vi "Main.vi"(8 "error in (no error)":errorcluster, 11 "ModuleAdmin":refnum<class "ModuleAdmin.lvclass">) -> ()   [LabVIEW 2018, in "MyPlugins.lvlib"]
uses:
  MyPlugins.lvlib
  <userlib>/NIST/ModuleAdminLib/ModuleAdmin/ModuleAdmin.lvclass
  C:/Program Files (x86)/National Instruments/LabVIEW 2018/user.lib/NIST/ModuleAdminLib/ModuleAdminBase/ModuleAdminBase.lvclass
  MyPluginBaseClass/MyPluginsBase.lvclass
  C:/Program Files (x86)/National Instruments/LabVIEW 2018/user.lib/NIST/BaseClasses/BasePlugin_class/BasePlugin.lvclass
  PluginsShared/clStopArgument.ctl
  <userlib>/NIST/ModuleAdminLib/ModuleAdmin/ModuleAdmin.lvclass/ModuleAdmin.ctl
  Queue SubVIs/DequeueTypes.ctl
  <userlib>/NIST/BaseClasses/BasePlugin_class/BasePlugin.lvclass/BasePlugin.ctl
  Queue SubVIs/EnqueueTypes.ctl
  <vilib>/Utility/error.llb/DialogType.ctl
  <userlib>/NIST/ModuleAdminLib/ModuleAdmin/Accessors/Read ShowPanel_.vi
  <userlib>/NIST/ModuleAdminLib/ModuleAdmin/Accessors/Write ShowPanel_.vi
  <userlib>/NIST/BaseClasses/BasePlugin_class/Accessors/Write PluginIniFilePath.vi
  <userlib>/NIST/BaseClasses/BasePlugin_class/Accessors/Read PluginIniFilePath.vi
  <userlib>/NIST/ModuleAdminLib/ModuleAdmin/Accessors/Read CloneRegRef.vi
  <vilib>/Utility/error.llb/Error Cluster From Error Code.vi
  <vilib>/ErrorRing/Error Ring.xnode
  <userlib>/NIST/ModuleAdminLib/CloneRegistration/CloneRegistration.lvclass
  PluginsShared/PluginsShared.lvlib
  <userlib>/NIST/BaseClasses/Object_class/BaseObject.lvclass
  <userlib>/NIST/ModuleAdminLib/ModuleAdmin.lvlib
panel:
  in  "USE FGV?":bool
  out "error out":errorcluster
  # "This is the template for your cloneable module.\nYou should modifiy this to perform the functionality\nthat you want it to perform"
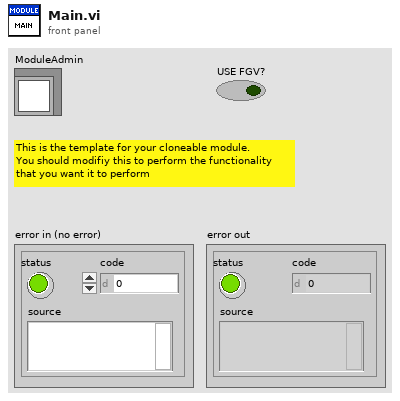
[diagram p1: front panel]
types:
  T1 = typedef "PluginsShared.lvlib/clRequestEvents.ctl" = cluster{"StopRequest":refnum<user-event>, "PathToINI":refnum<user-event>, " LoadPlugin":refnum<user-event>, "ShowPanel":refnum<user-event>, "PrefDlg":refnum<user-event>}
  T2 = typedef "PluginsShared.lvlib/clBroadcastEvents.ctl" = cluster{"DidInit":refnum<user-event>, "StatusUpdate":refnum<user-event>, "ErrorReport":refnum<user-event>, "DidStop":refnum<user-event>, "PathToINI":refnum<user-event>, "ReloadINIFiles":refnum<user-event>}
  T3 = typedef "PluginsShared.lvlib/clStopArgument.ctl" = cluster{"Exit via Stop Module Req?":bool, "Wait for Module to stop?":bool, "ModuleAdmin":refnum<class "ModuleAdmin.lvclass">}
  T4 = enum32{"Invalid", "Standard", "Closed", "Hidden", "Minimized", "Maximized"}
  T5 = typedef "MyPlugins.lvlib/EnqueueTypes.ctl" = enum16{"Enqueue", "Lossy Enqueue"}
  T6 = typedef "MyPlugins.lvlib/DequeueTypes.ctl" = enum16{"Dequeue", "Preview Queue"}
  T7 = typedef "DialogType.ctl" = u16
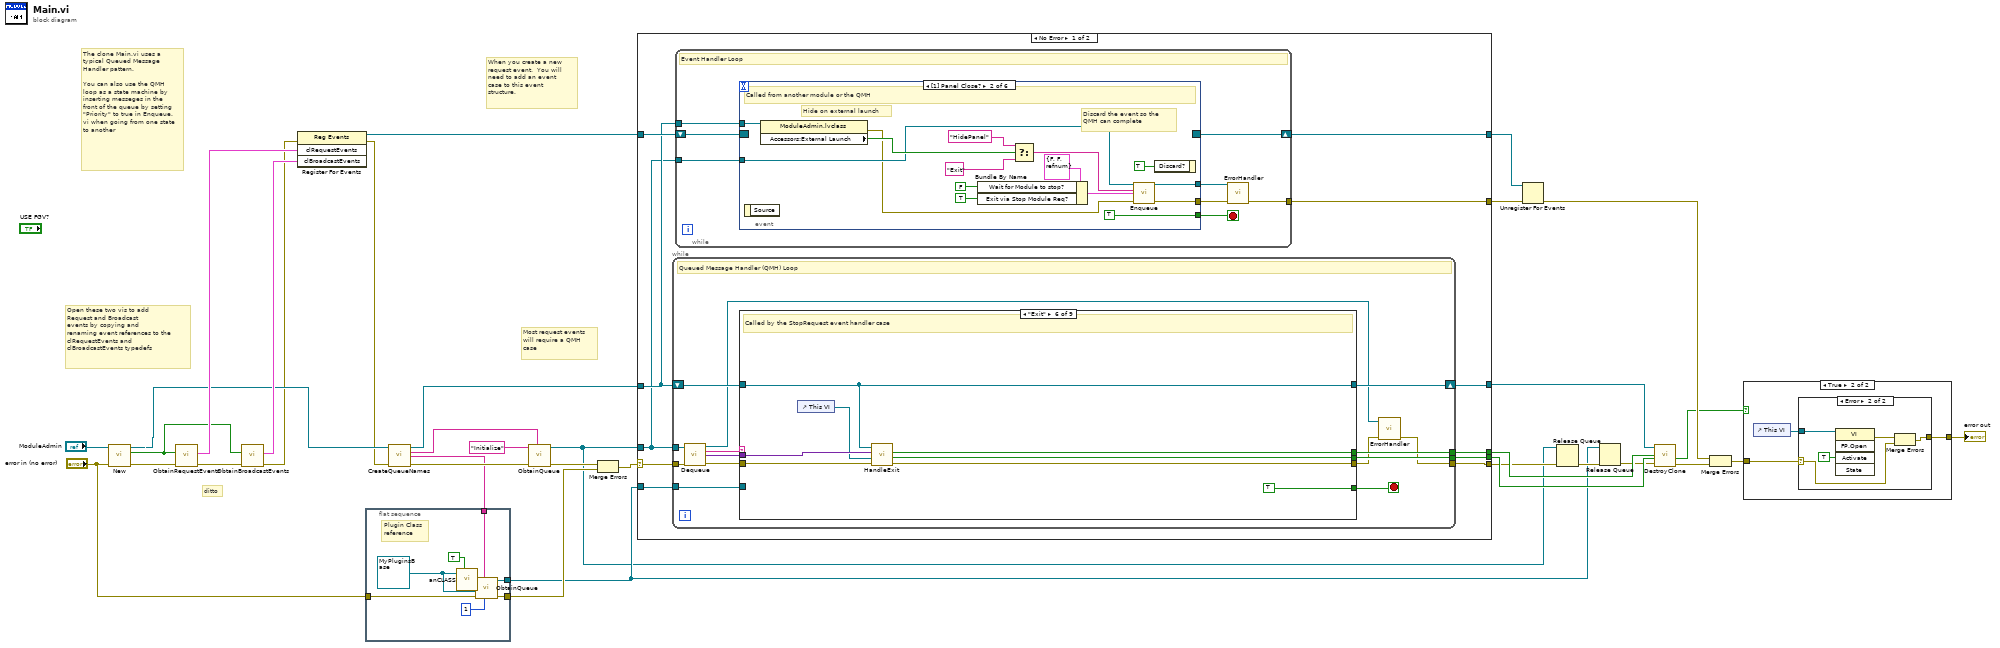
[diagram p0: block diagram]
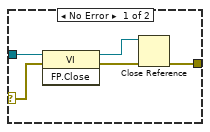
[diagram p3: hidden frame]
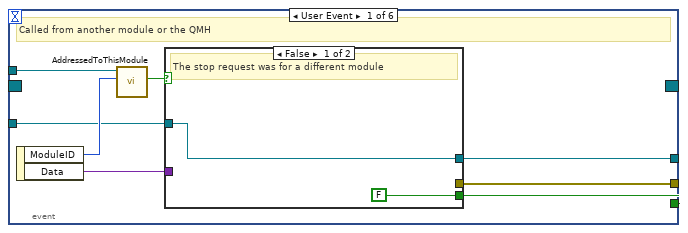
[diagram p4: hidden frame]
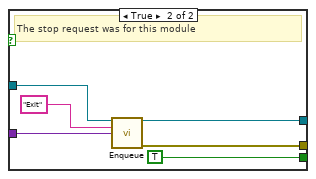
[diagram p5: hidden frame]
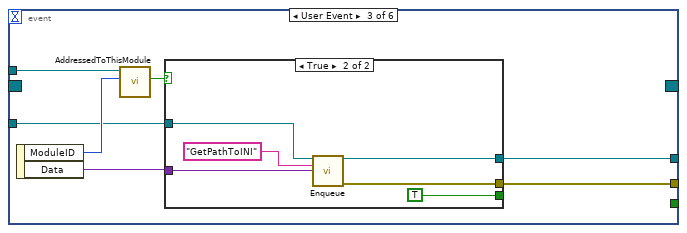
[diagram p6: hidden frame]
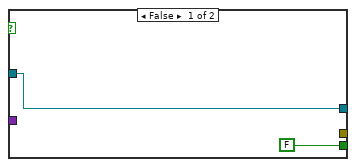
[diagram p7: hidden frame]
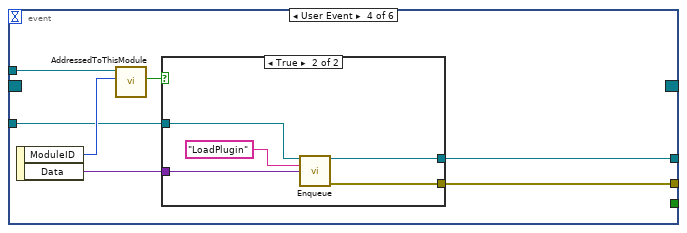
[diagram p8: hidden frame]
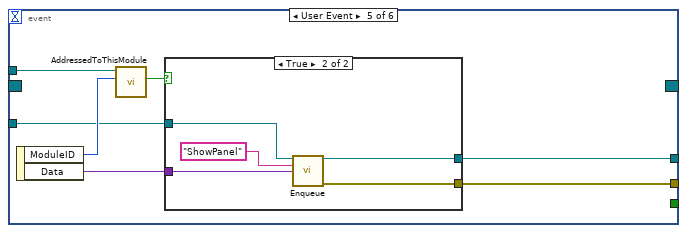
[diagram p10: hidden frame]
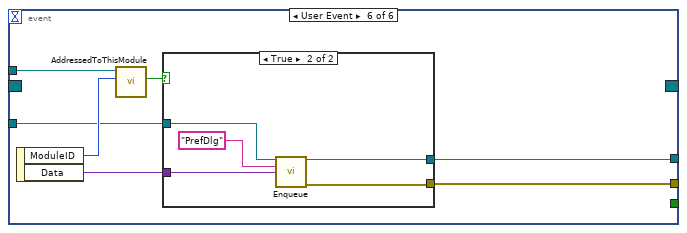
[diagram p12: hidden frame]
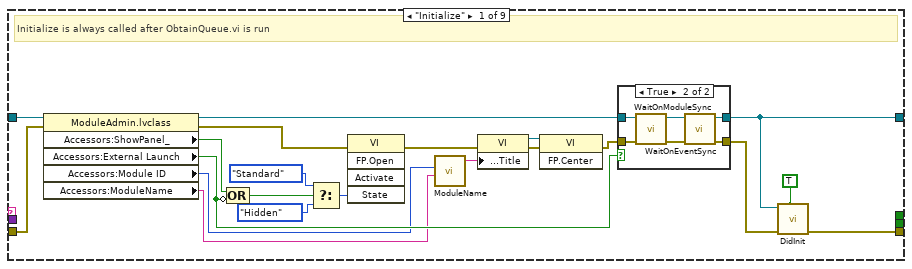
[diagram p14: hidden frame]
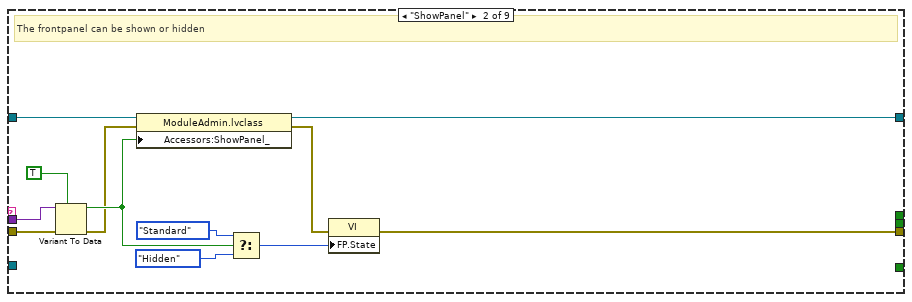
[diagram p16: hidden frame]
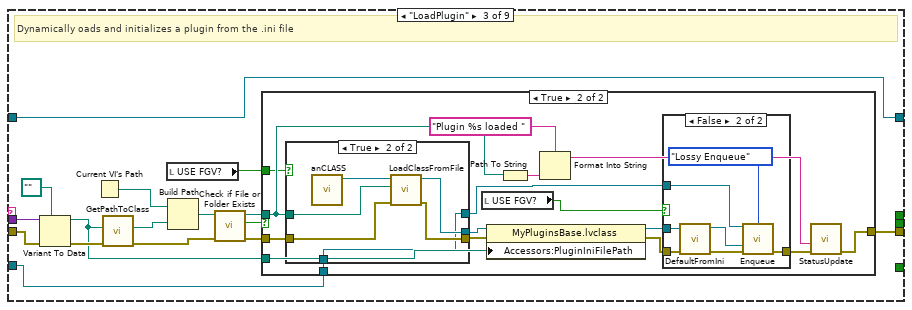
[diagram p17: hidden frame]
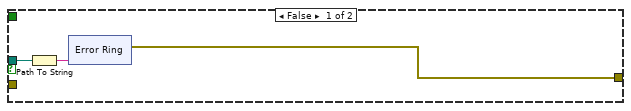
[diagram p18: hidden frame]
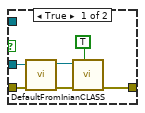
[diagram p19: hidden frame]
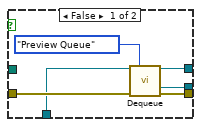
[diagram p20: hidden frame]
diagram:
  # "The clone Main.vi uses a typical Queued Message Handler pattern.  \n\nYou can also use the QMH loop as a state machine by inserting messeges in the front of the queue by setting \"Priority\" to true in Enqueue.vi when going from one state to another"
  # "Open these two vis to add\nRequest and Broadcast \nevents by copying and \nrenaming event references to the \nclRequestEvents and \nclBroadcastEvents typedefs"
  # "ditto"
  # "Most request events\nwill require a QMH\ncase"
  # "When you create a new request event.  You will need to add an event case to this event structure."
  n1 = call <userlib>:"New.vi"("error in (no error)"="error in (no error)", "ModuleAdmin"="ModuleAdmin") -> ("error out"=w25:errorcluster, "First?"=w32:bool, "ModuleAdmin"=w12:refnum<class "ModuleAdmin.lvclass">)  [unwired: 6 in, 1 out]
  n2 = call "ObtainRequestEvents.vi"("error in (no error)"=w25, "CreateNew (F)"=w32) -> ("error out"=w31:errorcluster, "clRequestEvents"=w33:T1)  [unwired: 8 in]
  n3 = call "ObtainBroadcastEvents.vi"("error in (no error)"=w31, "CreateNew? (F)"=w32) -> ("error out"=w6:errorcluster, "clBroadcastEvents"=w30:T2)  [unwired: 8 in]
  n4 = register-events(error in=w6, w33, w30) -> (reference out=w29:refnum<event-registration>, error out=w5:errorcluster)  [unwired: 1 in]
  n5 = flat-sequence {
    tunnel: "error in (no error)" -> [w40]
    tunnel: [w39] -> w22
    tunnel: w8 -> [w38]
    tunnel: [w36] -> w2
    frame #0 {
      w37 = refnum<class "MyPluginsBase.lvclass"> refnum ("MyPlugins.lvlib:MyPluginsBase.lvclass")
      # "Plugin Class\nreference"
      n6 = call "anCLASS.vi"("Set? (f)"=TRUE, "MyPlugins.lvlib In"=w37) -> ()  [unwired: 9 in, 1 out]
      n7 = call "ObtainQueue.vi"("max queue size (-1, unlimited)"=1, "Queue Name"=w38, "Error In"=w40, "MyPluginsClass"=w37) -> ("Error Out"=w39:errorcluster, "queue out"=w36:refnum<queue>)  [unwired: 6 in]
    }
  }
  n8 = call "CreateQueueNames.vi"("ModuleAdmin"=w12, "error in (no error)"=w5) -> ("ModuleAdmin Out"=w10:refnum<class "ModuleAdmin.lvclass">, "QMH Queue Name"=w9:string, "Class Queue Name"=w8:string, "error out"=w11:errorcluster)  [unwired: 9 in, 1 out]
  n9 = call "ObtainQueue.vi"("Queue Name"=w9, "Error In"=w11, "InitialMessage"="Initialize" ("Message")) -> ("Error Out"=w14:errorcluster, "queue out"=w1:refnum<queue>)  [unwired: 7 in]
  n10 = Merge Errors(w14, w22) -> (w23:errorcluster)
  n11 = case shown="No Error" w23 {
    selector: w23 -> [w52 w376]
    tunnel: w10 -> [w45 w369]
    tunnel: [w44 w374] -> w16
    tunnel: w29 -> [w51 w370]
    tunnel: [w50 w373] -> w7
    tunnel: [w49 _] -> w19
    tunnel: [w48 _] -> w18
    tunnel: [w47 _] -> w28
    tunnel: [w46 w370] -> w27
    tunnel: w1 -> [w43 _]
    tunnel: w2 -> [w42 _]
    frame No Error {
      n12 = while {
        tunnel: w52 -> [w158]
        tunnel: [w152] -> w44
        tunnel: [w154] -> w49
        tunnel: [w153] -> w48
        shift-right: [w148] -> w50
        shift-left: w45 -> [w149]
        tunnel: w43 -> [w150]
        tunnel: w42 -> [w147]
        stop <- w159 stop-if-true
        # "Queued Message Handler (QMH) Loop"
        n13 = call "Dequeue.vi"("queue in"=w150, "error in (no error)"=w158) -> ("queue out"=w146:refnum<queue>, "Message"=w156:string, "Message Data"=w155:variant, "error out"=w157:errorcluster)  [unwired: 9 in, 1 out]
        n14 = case shown="\"Exit\"" w156 {
          selector: w156 -> [_ _ _ _ _ _ _ _ w357]
          tunnel: [_ _ _ _ _ TRUE _ TRUE _] -> w159
          tunnel: [w170 w193 w205 w275 w293 w329 w332 w349 w351] -> w151
          tunnel: w157 -> [w164 w200 w214 w273 w295 w328 w340 _ _]
          tunnel: w155 -> [_ w199 w216 _ _ w327 w339 _ _]
          tunnel: [_ _ _ _ _ w325 _ _ _] -> w154
          tunnel: [_ _ _ _ _ w324 _ _ _] -> w153
          tunnel: w149 -> [w161 w192 w201 w270 w291 w323 w331 w345 w355]
          tunnel: [w160 w189 w201 w269 w290 w323 w331 w345 w354] -> w148
          tunnel: w147 -> [_ _ w202 w267 w288 _ _ _ _]
          frame "Initialize" {
            # "Initialize is always called after ObtainQueue.vi is run"
            n15 = property class="ModuleAdmin.lvclass"(reference=w161, error in=w164) -> (reference out=w168:refnum<class "ModuleAdmin.lvclass">, error out=w178:errorcluster, "Accessors:ShowPanel_"=w167:bool, "Accessors:External Launch"=w166:bool, "Accessors:Module ID"=w162:i32, "Accessors:ModuleName"=w163:string)
            n16 = Compound Arithmetic op=OR(w167, invert w166) -> (w165:bool)
            n17 = Select(t=T4."Standard" ("Front Panel Window:State"), s=w165, f=T4."Hidden" ("Front Panel Window:State")) -> (s? t:f=w174:T4)
            n18 = invoke class="VI" method="FP.Open"(error in=w178, "State"=w174) -> (error out=w177:errorcluster)  [unwired: 3 in, 4 out]
            n19 = call <userlib>:"ModuleName.vi"("Name"=w163, "ModuleID"=w162) -> ("ModuleName"=w173:string)  [unwired: 9 in]
            n20 = property class="VI"(error in=w177, "Front Panel.Title"=w173) -> (reference out=w180:refnum<vi>, error out=w179:errorcluster)  [unwired: 1 in]
            n21 = invoke class="VI" method="FP.Center"(reference=w180, error in=w179) -> (error out=w169:errorcluster)  [unwired: 1 in, 2 out]
            n22 = case shown="True" w166 {
              tunnel: [w181 w187] -> w171
              tunnel: [w182 w184] -> w160
              tunnel: w169 -> [w181 w186]
              tunnel: w168 -> [w182 w183]
              frame False {
              }
              frame True {
                n23 = call <userlib>:"WaitOnModuleSync.vi"("error in (no error)"=w186, "ModuleAdmin"=w183) -> ("error out"=w188:errorcluster, "ModuleAdmin"=w185:refnum<class "ModuleAdmin.lvclass">)  [unwired: 8 in]
                n24 = call <userlib>:"WaitOnEventSync.vi"("error in (no error)"=w188, "ModuleAdmin"=w185) -> ("error out"=w187:errorcluster, "ModuleAdmin"=w184:refnum<class "ModuleAdmin.lvclass">)  [unwired: 8 in]
              }
            }
            n25 = call "DidInit.vi"("Init?"=TRUE, "error in (no error)"=w171, "ModuleAdmin"=w160) -> ("error out"=w170:errorcluster)  [unwired: 8 in]
          }
          frame "ShowPanel" {
            # "The frontpanel can be shown or hidden"
            n26 = Variant To Data(error in=w200, type=TRUE, Variant=w199) -> (data=w195:bool, error out=w191:errorcluster)
            n27 = property class="ModuleAdmin.lvclass"(reference=w192, error in=w191, "Accessors:ShowPanel_"=w195) -> (reference out=w189:refnum<class "ModuleAdmin.lvclass">, error out=w190:errorcluster)
            n28 = Select(t=T4."Standard" ("Front Panel Window:State"), s=w195, f=T4."Hidden" ("Front Panel Window:State")) -> (s? t:f=w194:T4)
            n29 = property class="VI"(error in=w190, "FP.State"=w194) -> (error out=w193:errorcluster)  [unwired: 1 in, 1 out]
          }
          frame "LoadPlugin" {
            # "Dynamically oads and initializes a plugin from the .ini file"
            n30 = Variant To Data(error in=w214, type=path "", Variant=w216) -> (data=w204:path, error out=w213:errorcluster)
            n31 = Current VI's Path() -> (path=w211:path)
            n32 = call <userlib>:"GetPathToClass.vi"("error in (no error)"=w213, "configuration file path"=w204) -> ("error IO"=w209:errorcluster, "PathToClass"=w212:path)  [unwired: 8 in]
            n33 = local read "USE FGV?"() -> (w203:bool)
            n34 = Build Path(base path=w211, name or relative path=w212) -> (appended path=w210:path)
            n35 = call <vilib>:"Check if File or Folder Exists.vi"("error in (no error)"=w209, "path"=w210) -> ("error out"=w206:errorcluster, "file or folder exists?"=w208:bool, "dup path"=w207:path)  [unwired: 7 in]
            n36 = case shown="True" w208 {
              tunnel: w207 -> [w218 w236]
              tunnel: w206 -> [_ w242]
              tunnel: [w217 w238] -> w205
              tunnel: w204 -> [_ w234]
              tunnel: w203 -> [_ w230]
              tunnel: w202 -> [_ w229]
              frame False {
                n37 = Path To String(path=w218) -> (string=w219:string)
                n38 = xnode "Error Ring"("parameter 0"=w219) -> ("error out"=w217:errorcluster)
              }
              frame True {
                n39 = case shown="True" w230 {
                  tunnel: w242 -> [w260 w266]
                  tunnel: [w258 w265] -> w237
                  tunnel: w236 -> [_ w264]
                  tunnel: [w259 w263] -> w235
                  tunnel: w229 -> [w257 w261]
                  tunnel: [w255 w261] -> w227
                  frame False {
                    n40 = call "Dequeue.vi"("queue in"=w257, "Dequeue Type"=DequeueTypes."Preview Queue", "error in (no error)"=w260) -> ("queue out"=w255:refnum<queue>, "MyPluginsClass"=w258:refnum<class "MyPluginsBase.lvclass">, "error out"=w259:errorcluster)  [unwired: 8 in, 2 out]
                  }
                  frame True {
                    n41 = call "anCLASS.vi"() -> ("MyPlugins.lvlib Out"=w262:refnum<class "MyPluginsBase.lvclass">)  [unwired: 11 in]
                    n42 = call-dynamic "LoadClassFromFile.vi"("error in (no error)"=w266, "class path"=w264, "reference in"=w262) -> ("error out"=w263:errorcluster, "reference out"=w265:refnum<class "MyPluginsBase.lvclass">)  [unwired: 7 in]
                  }
                }
                n43 = local read "USE FGV?"() -> (w228:bool)
                n44 = property class="MyPluginsBase.lvclass"(reference=w237, error in=w235, "Accessors:PluginIniFilePath"=w234) -> (reference out=w233:refnum<class "MyPluginsBase.lvclass">, error out=w232:errorcluster)
                n45 = Path To String(path=w236) -> (string=w240:string)
                n46 = Format Into String(format string="Plugin %s loaded ", w240) -> (resulting string=w239:string)  [unwired: 2 in, 1 out]
                n47 = case shown="False" w228 {
                  tunnel: w233 -> [w247 w254]
                  tunnel: w232 -> [w246 w253]
                  tunnel: [w245 w250] -> w231
                  tunnel: w227 -> [_ w248]
                  frame True {
                    n48 = call-dynamic "DefaultFromIni.vi"("error in (no error)"=w246, "MyPluginsBase in"=w247) -> ("error out"=w245:errorcluster, "MyPluginsBase out"=w244:refnum<class "MyPluginsBase.lvclass">)  [unwired: 8 in]
                    n49 = call "anCLASS.vi"("Set? (f)"=TRUE, "MyPlugins.lvlib In"=w244) -> ()  [unwired: 9 in, 1 out]
                  }
                  frame False {
                    n50 = call-dynamic "DefaultFromIni.vi"("error in (no error)"=w253, "MyPluginsBase in"=w254) -> ("error out"=w251:errorcluster, "MyPluginsBase out"=w252:refnum<class "MyPluginsBase.lvclass">)  [unwired: 8 in]
                    n51 = call "Enqueue.vi"("queue in"=w248, "Enqueue Type (Enqueue)"=EnqueueTypes."Lossy Enqueue", "MyPluginsClass"=w252, "error in (no error)"=w251) -> ("error out"=w250:errorcluster)  [unwired: 10 in, 1 out]
                  }
                }
                n52 = call "StatusUpdate.vi"("error in (no error)"=w231, "Status"=w239) -> ("error out"=w238:errorcluster)  [unwired: 8 in, 1 out]
              }
            }
          }
          frame "GetPathToINI" {
            # "Broadcast the path to the .ini file"
            n53 = local read "USE FGV?"() -> (w268:bool)
            n54 = case shown="False" w268 {
              tunnel: [w280 w287] -> w274
              tunnel: w273 -> [w279 w285]
              tunnel: [w277 w286] -> w272
              tunnel: w267 -> [_ w282]
              frame True {
                n55 = call "anCLASS.vi"() -> ("MyPlugins.lvlib Out"=w278:refnum<class "MyPluginsBase.lvclass">)  [unwired: 11 in]
                n56 = property class="MyPluginsBase.lvclass"(reference=w278, error in=w279) -> (error out=w277:errorcluster, "Accessors:PluginIniFilePath"=w280:path)  [unwired: 1 out]
              }
              frame False {
                n57 = call "Dequeue.vi"("queue in"=w282, "Dequeue Type"=DequeueTypes."Preview Queue", "error in (no error)"=w285) -> ("MyPluginsClass"=w283:refnum<class "MyPluginsBase.lvclass">, "error out"=w284:errorcluster)  [unwired: 8 in, 3 out]
                n58 = property class="MyPluginsBase.lvclass"(reference=w283, error in=w284) -> (error out=w286:errorcluster, "Accessors:PluginIniFilePath"=w287:path)  [unwired: 1 out]
              }
            }
            n59 = property class="ModuleAdmin.lvclass"(reference=w270, error in=w272) -> (reference out=w269:refnum<class "ModuleAdmin.lvclass">, error out=w271:errorcluster, "Accessors:Module ID"=w276:i32)
            n60 = call "PathToINIBroadcast.vi"("error in (no error)"=w271, "PathToINI"=w274, "ModuleID"=w276) -> ("error out"=w275:errorcluster)  [unwired: 8 in]
          }
          frame "PrefDlg" {
            # "Override Base Class\\PublicMethods\\PrefDialog.vi for user editable preference dialog"
            # "Launch the modal Preferences dialog"
            n61 = local read "USE FGV?"() -> (w289:bool)
            n62 = case shown="False" w289 {
              tunnel: w295 -> [w308 w314]
              tunnel: [w304 w312] -> w294
              tunnel: [w302 w310] -> w292
              tunnel: w288 -> [w307 _]
              frame False {
                n63 = call "Dequeue.vi"("queue in"=w307, "Dequeue Type"=DequeueTypes."Preview Queue", "error in (no error)"=w308) -> ("queue out"=w301:refnum<queue>, "MyPluginsClass"=w297:refnum<class "MyPluginsBase.lvclass">, "error out"=w306:errorcluster)  [unwired: 8 in, 2 out]
                n64 = call-dynamic "PrefDialog.vi"("error in (no error)"=w306, "MyPluginsBase in"=w297) -> ("error out"=w303:errorcluster, "ReloadiniFiles"=w304:bool, "ChangeOccured?"=w299:bool, "MyPluginsBase out"=w298:refnum<class "MyPluginsBase.lvclass">)  [unwired: 6 in]
                n65 = Select(t=w298, s=w299, f=w297) -> (s? t:f=w296:refnum<class "MyPluginsBase.lvclass">)
                n66 = call "Enqueue.vi"("queue in"=w301, "Enqueue Type (Enqueue)"=EnqueueTypes."Lossy Enqueue", "MyPluginsClass"=w296, "error in (no error)"=w303) -> ("error out"=w302:errorcluster)  [unwired: 10 in, 1 out]
              }
              frame True {
                n67 = call "anCLASS.vi"() -> ("MyPlugins.lvlib Out"=w313:refnum<class "MyPluginsBase.lvclass">)  [unwired: 11 in]
                n68 = call-dynamic "PrefDialog.vi"("error in (no error)"=w314, "MyPluginsBase in"=w313) -> ("error out"=w310:errorcluster, "ReloadiniFiles"=w312:bool, "ChangeOccured?"=w309:bool, "MyPluginsBase out"=w311:refnum<class "MyPluginsBase.lvclass">)  [unwired: 6 in]
                n69 = call "anCLASS.vi"("Set? (f)"=w309, "MyPlugins.lvlib In"=w311) -> ()  [unwired: 9 in, 1 out]
              }
            }
            n70 = case shown="True" w294 {
              tunnel: [w316 w322] -> w293
              tunnel: w292 -> [w316 w319]
              tunnel: w291 -> [w315 w318]
              tunnel: [w315 w317] -> w290
              frame False {
              }
              frame True {
                n71 = property class="ModuleAdmin.lvclass"(reference=w318, error in=w319) -> (reference out=w317:refnum<class "ModuleAdmin.lvclass">, error out=w321:errorcluster, "Accessors:Module ID"=w320:i32)
                n72 = call "ReloadINIFiles.vi"("error in (no error)"=w321, "ModuleID"=w320) -> ("error out"=w322:errorcluster)  [unwired: 9 in]
              }
            }
          }
          frame "Exit" {
            # "Called by the StopRequest event handler case"
            n73 = control-ref of="This VI"() -> (w326:refnum<vi>)
            n74 = call "HandleExit.vi"("error in (no error)"=w328, "VI Refnum"=w326, "StopArgument"=w327, "ModuleAdmin"=w323) -> ("error out"=w329:errorcluster, "Exit via Stop Module Req?"=w324:bool, "WaitForStop?"=w325:bool)  [unwired: 5 in]
          }
          frame "Error" {
            # "Handle any errors"
            n75 = property class="ModuleAdmin.lvclass"(reference=w331) -> ("Accessors:External Launch"=w335:bool, "Accessors:Module ID"=w333:i32)  [unwired: 1 in, 2 out]
            n76 = Variant To Data(error in=w340, type=errorcluster {"status"=FALSE, "code"=0, "source"=""} ("error constant"), Variant=w339) -> (data=w334:errorcluster, error out=w337:errorcluster)
            n77 = call "ReportError.vi"("error in (no error)"=w337, "ErrorReported"=w334, "ModuleID"=w333) -> ("error out"=w336:errorcluster)  [unwired: 8 in]
            n78 = case shown="True" w335 {
              tunnel: w336 -> [w343 w344]
              tunnel: w334 -> [w342 _]
              tunnel: [w341 w344] -> w332
              frame False {
                # "Todo:  Add an event to ask the user\nIf the module should stop or continue"
                # "Stand alone: now, force an exit"
                n79 = call <vilib>:"Simple Error Handler.vi"("error in (no error)"=w342) -> ()  [unwired: 4 in, 5 out]
                n80 = call "StopRequest.vi"("error in (no error)"=w343) -> ("error out"=w341:errorcluster)  [unwired: 9 in, 1 out]
              }
              frame True {
                # "Externally launched modules only broadcast the error msg"
              }
            }
          }
          frame "QueueError" {
            n81 = call "StatusUpdate.vi"("Status"=" Queue Error" ("format string"), "Module"=w345) -> ("error out"=w350:errorcluster, "Module"=w348:refnum<class "ModuleAdmin.lvclass">)  [unwired: 8 in]
            n82 = call "StopRequest.vi"("error in (no error)"=w350, "ModuleAdmin"=w348) -> ("error out"=w349:errorcluster)  [unwired: 8 in, 1 out]
          }
          frame Default {
            # "Called only if a message was queued and no QMH case was created"
            n83 = property class="ModuleAdmin.lvclass"(reference=w355) -> (reference out=w354:refnum<class "ModuleAdmin.lvclass">, error out=w352:errorcluster, "Accessors:Module ID"=w359:i32, "Accessors:ModuleName"=w356:string)  [unwired: 1 in]
            n84 = call <userlib>:"ModuleName.vi"("Name"=w356, "ModuleID"=w359) -> ("ModuleName"=w358:string)  [unwired: 9 in]
            n85 = xnode "Error Ring"("parameter 0"=w357, "parameter 1"=w358) -> ("error out"=w353:errorcluster)
            n86 = Merge Errors(w352, w353) -> (w351:errorcluster)
          }
        }
        n87 = call "ErrorHandler.vi"("error in (no error)"=w151, "queue in"=w146) -> ("error out"=w152:errorcluster)  [unwired: 8 in, 1 out]
      }
      n88 = while {
        tunnel: w45 -> [w55]
        shift-right: [w58] -> w46
        shift-left: w51 -> [w59]
        tunnel: [w56] -> w47
        tunnel: w43 -> [w54]
        stop <- w60 stop-if-true
        # "Event Handler Loop"
        n89 = event shown="[1] Panel Close?" {
          selector: w59 -> [_ _ _ _ _ _]
          dyn-events: [_ _ _ _ _ _] -> w58
          timeout: _ -> [_ _ _ _ _ _]
          tunnel: w55 -> [w63 w81 w94 w109 w122 w135]
          tunnel: [w66 TRUE _ _ _ _] -> w60
          tunnel: [w65 w90 w95 w111 w124 w137] -> w57
          tunnel: w54 -> [w62 w79 w93 w108 w121 w134]
          tunnel: [w61 w80 w92 w107 w120 w133] -> w53
          event User Event {
            # "Called from another module or the QMH"
            n90 = event-data() -> ("ModuleID"=w67:i32, "Data"=w64:variant)  [unwired: 1 in]
            n91 = call <userlib>:"AddressedToThisModule.vi"("ModuleID"=w67, "ModuleAdmin"=w63) -> ("AddressedToThisInstance?"=w68:bool)  [unwired: 8 in, 1 out]
            n92 = case shown="False" w68 {
              tunnel: [FALSE TRUE] -> w66
              tunnel: [_ w75] -> w65
              tunnel: w64 -> [_ w73]
              tunnel: w62 -> [w69 w72]
              tunnel: [w69 w71] -> w61
              frame False {
                # "The stop request was for a different module"
              }
              frame True {
                # "The stop request was for this module"
                n93 = call "Enqueue.vi"("queue in"=w72, "Message"="Exit", "Message Data"=w73) -> ("queue out"=w71:refnum<queue>, "error out"=w75:errorcluster)  [unwired: 11 in]
              }
            }
          }
          event Panel Close? {
            # "Hide on external launch"
            # "Discard the event so the QMH can complete"
            # "Called from another module or the QMH"
            n94 = event-data() -> ()  [unwired: 1 in, 1 out]
            n95 = property class="ModuleAdmin.lvclass"(reference=w81) -> (error out=w78:errorcluster, "Accessors:External Launch"=w82:bool)  [unwired: 1 in, 1 out]
            n96 = Bundle By Name(cluster=T3 {"Exit via Stop Module Req?"=FALSE, "Wait for Module to stop?"=FALSE, "ModuleAdmin"=refnum} ("Stop Argument"), "Wait for Module to stop?"=FALSE, "Exit via Stop Module Req?"=TRUE) -> (w87:T3)
            n97 = Select(t="HidePanel", s=w82, f="Exit" ("Message")) -> (s? t:f=w84:string)
            n98 = call "Enqueue.vi"("queue in"=w79, "Message"=w84, "Message Data"=w87, "error in (no error)"=w78) -> ("queue out"=w80:refnum<queue>, "error out"=w90:errorcluster)  [unwired: 10 in]
            n99 = event-data("Discard?"=TRUE) -> ()  [unwired: 1 in, 1 out]
          }
          event User Event {
            n100 = event-data() -> ("ModuleID"=w96:i32, "Data"=w97:variant)  [unwired: 1 in]
            n101 = call <userlib>:"AddressedToThisModule.vi"("ModuleID"=w96, "ModuleAdmin"=w94) -> ("AddressedToThisInstance?"=w98:bool)  [unwired: 8 in, 1 out]
            n102 = case shown="True" w98 {
              tunnel: [FALSE TRUE] -> _
              tunnel: [_ w105] -> w95
              tunnel: w97 -> [_ w103]
              tunnel: w93 -> [w99 w102]
              tunnel: [w99 w101] -> w92
              frame False {
                # "The stop request was for a different module"
              }
              frame True {
                # "The stop request was for this module"
                n103 = call "Enqueue.vi"("queue in"=w102, "Message"="GetPathToINI", "Message Data"=w103) -> ("queue out"=w101:refnum<queue>, "error out"=w105:errorcluster)  [unwired: 11 in]
              }
            }
          }
          event User Event {
            n104 = event-data() -> ("ModuleID"=w113:i32, "Data"=w110:variant)  [unwired: 1 in]
            n105 = call <userlib>:"AddressedToThisModule.vi"("ModuleID"=w113, "ModuleAdmin"=w109) -> ("AddressedToThisInstance?"=w112:bool)  [unwired: 8 in, 1 out]
            n106 = case shown="True" w112 {
              tunnel: [_ w117] -> w111
              tunnel: w110 -> [_ w118]
              tunnel: w108 -> [w114 w116]
              tunnel: [w114 w115] -> w107
              frame False {
              }
              frame True {
                n107 = call "Enqueue.vi"("queue in"=w116, "Message"="LoadPlugin", "Message Data"=w118) -> ("queue out"=w115:refnum<queue>, "error out"=w117:errorcluster)  [unwired: 11 in]
              }
            }
          }
          event User Event {
            n108 = event-data() -> ("ModuleID"=w126:i32, "Data"=w123:variant)  [unwired: 1 in]
            n109 = call <userlib>:"AddressedToThisModule.vi"("ModuleID"=w126, "ModuleAdmin"=w122) -> ("AddressedToThisInstance?"=w125:bool)  [unwired: 8 in, 1 out]
            n110 = case shown="True" w125 {
              tunnel: [_ w130] -> w124
              tunnel: w123 -> [_ w131]
              tunnel: w121 -> [w127 w129]
              tunnel: [w127 w128] -> w120
              frame False {
              }
              frame True {
                n111 = call "Enqueue.vi"("queue in"=w129, "Message"="ShowPanel", "Message Data"=w131) -> ("queue out"=w128:refnum<queue>, "error out"=w130:errorcluster)  [unwired: 11 in]
              }
            }
          }
          event User Event {
            n112 = event-data() -> ("ModuleID"=w139:i32, "Data"=w136:variant)  [unwired: 1 in]
            n113 = call <userlib>:"AddressedToThisModule.vi"("ModuleID"=w139, "ModuleAdmin"=w135) -> ("AddressedToThisInstance?"=w138:bool)  [unwired: 8 in, 1 out]
            n114 = case shown="True" w138 {
              tunnel: [_ w143] -> w137
              tunnel: w136 -> [_ w144]
              tunnel: w134 -> [w140 w142]
              tunnel: [w140 w141] -> w133
              frame False {
              }
              frame True {
                n115 = call "Enqueue.vi"("queue in"=w142, "Message"="PrefDlg", "Message Data"=w144) -> ("queue out"=w141:refnum<queue>, "error out"=w143:errorcluster)  [unwired: 11 in]
              }
            }
          }
        }
        n116 = call "ErrorHandler.vi"("error in (no error)"=w57, "queue in"=w53) -> ("error out"=w56:errorcluster)  [unwired: 8 in, 1 out]
      }
    }
    frame Error {
      n117 = property class="ModuleAdmin.lvclass"(reference=w369) -> (reference out=w373:refnum<class "ModuleAdmin.lvclass">, error out=w368:errorcluster, "Accessors:CloneRegRef"=w372:refnum<data-value>, "Accessors:Module ID"=w371:i32)  [unwired: 1 in]
      n118 = call <userlib>:"Remove.vi"("error in (no error)"=w368, "Module ID"=w371, "CloneRegRef"=w372) -> ("error out"=w375:errorcluster)  [unwired: 6 in, 2 out]
      n119 = flat-sequence {
        tunnel: w376 -> [w381]
        tunnel: w375 -> [w377]
        tunnel: [w379] -> w374
        frame #0 {
          w380 = T7 2 items=["no dialog", "OK message", "continue or stop message", "OK message + warnings", "continue/stop + warnings"] ("type of dialog (OK msg:1)")
          n120 = Merge Errors(w377, w381) -> (w378:errorcluster)
          n121 = call <vilib>:"Simple Error Handler.vi"("type of dialog (OK msg:1)"=w380, "error in (no error)"=w378) -> ("error out"=w379:errorcluster)  [unwired: 3 in, 4 out]
        }
      }
    }
  }
  n122 = Unregister For Events(event registration refnum=w27, error in=w28) -> (error out=w26:errorcluster)
  n123 = Release Queue(queue=w1, error in (no error)=w16) -> (error out=w4:errorcluster)  [unwired: 1 in, 2 out]
  n124 = Release Queue(queue=w2, error in (no error)=w4) -> (error out=w3:errorcluster)  [unwired: 1 in, 2 out]
  n125 = call "DestroyClone.vi"("error in (no error)"=w3, "Exit via Stop Module Req?"=w18, "Wait for Module to stop?"=w19, "ModuleAdmin"=w7) -> ("error out"=w20:errorcluster, "External Launch"=w17:bool)  [unwired: 5 in, 1 out]
  n126 = Merge Errors(w26, w20) -> (w21:errorcluster)
  n127 = case shown="True" w17 {
    tunnel: w21 -> [w382 w385]
    tunnel: [w382 w383] -> w15
    frame False {
    }
    frame True {
      n128 = control-ref of="This VI"() -> (w384:refnum<vi>)
      n129 = case shown="Error" w385 {
        selector: w385 -> [w389 w393]
        tunnel: w384 -> [w390 w394]
        tunnel: [w386 w392] -> w383
        frame No Error {
          n130 = invoke class="VI" method="FP.Close"(reference=w390, error in=w389) -> (reference out=w387:refnum<vi>, error out=w388:errorcluster)  [unwired: 1 in, 1 out]
          n131 = Close Reference(reference=w387, error in (no error)=w388) -> (error out=w386:errorcluster)
        }
        frame Error {
          n132 = invoke class="VI" method="FP.Open"(reference=w394, "Activate"=TRUE ("Activate?")) -> (error out=w391:errorcluster)  [unwired: 3 in, 4 out]
          n133 = Merge Errors(w391, w393) -> (w392:errorcluster)
        }
      }
    }
  }
  "error out" <- w15
